vi "TimeArrayToTimestampInfo.vi"(8 "Units":enum16{"Miliseconds", "Seconds"}(ring), 9 "Append":string, 10 "Number of iterations":dbl=1.0 min=1.0, 11 "Times array in":refnum<vi>[](array[refnum])) -> (3 "Array out":string[](array[string]))   [LabVIEW 2017]
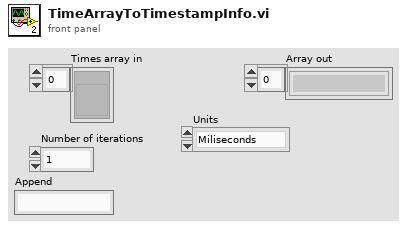
[diagram p1: front panel]
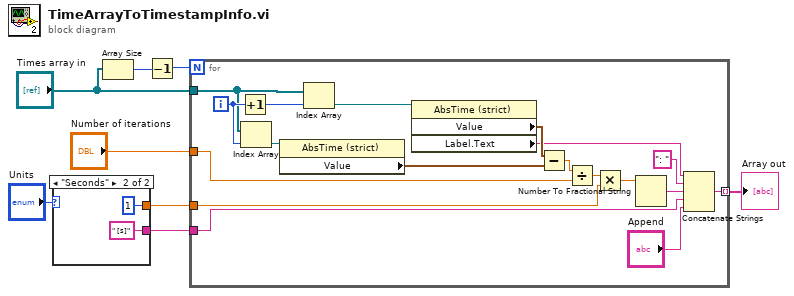
[diagram p0: block diagram]
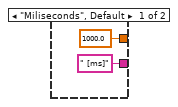
[diagram p2: hidden frame]
diagram:
  n1 = case shown="\"Seconds\"" "Units" {
    tunnel: [1000.0 1] -> w1
    tunnel: [" [ms]" " [s]"] -> w2
    frame "Miliseconds", Default {
    }
    frame "Seconds" {
    }
  }
  n2 = Array Size(array="Times array in") -> (size(s)=w4:i32)
  n3 = Decrement(x=w4) -> (x-1=w5:i32)
  n4 = for {
    N: w5 -> [_]
    tunnel: "Times array in" -> [w23]
    tunnel: [w28] -> w7 mode=indexing
    tunnel: "Number of iterations" -> [w25]
    tunnel: w2 -> [w16]
    tunnel: w1 -> [w14]
    i -> [w30]
    n5 = Increment(x=w30) -> (x+1=w24:i32)
    n6 = Index Array(array=w23, index=w30) -> (element=w22:refnum<vi>)
    n7 = property class="AbsTime (strict)"(reference=w22) -> ("Value"=w19:timestamp)  [unwired: 1 in, 2 out]
    n8 = Index Array(array=w23, index=w24) -> (element=w21:refnum<vi>)
    n9 = property class="AbsTime (strict)"(reference=w21) -> ("Value"=w20:timestamp, "Label.Text"=w18:string)  [unwired: 1 in, 2 out]
    n10 = Subtract(x=w20, y=w19) -> (x-y=w26:dbl)
    n11 = Divide(x=w26, y=w25) -> (x/y=w15:dbl)
    n12 = Multiply(x=w15, y=w14) -> (x*y=w13:dbl)
    n13 = Number To Fractional String(number=w13) -> (F-format string=w27:string)  [unwired: 3 in]
    n14 = Concatenate Strings(w18, ": " ("string"), w27, w16, "Append") -> (w28:string)
  }
  "Array out" <- w7
